vi "init.vi"(3 "Container State":T11, 4 "Previous State":variant, 5 "Previous Version":T10) -> (2 "Current State":T1={"current frame index"=0, "number of images"=0, "ROI (frames)"={"ROI"=[]}, "control refs"={"frame"=refnum, "image"=refnum, "saveROIsButton"=refnum, "loadImageSwitch"=refnum, "loadROIsSwitch"=refnum, "saveROIsSwitch"=refnum, "loadImagePath"=refnum, "loadROIPath"=refnum, "redraw"=refnum}, "calibration"={"x"=0.0, "y"=0.0, "x unit"=enum."um", "y unit"=enum."um"}, "xpaths"={"x offset"="", "y offset"="", "z offset"=""}, "offset"=refnum, "XML description"="", "number of ROIs"=0.0, "ROI Tool Buttons Visible"={"Zoom Tool"=FALSE, "Selection Tool"=FALSE, "Pan Tool"=FALSE, "Point Tool"=FALSE, "Line Tool"=FALSE, "Rectangle Tool"=FALSE, "Rotated Rectangle Tool"=FALSE, "Polyline Tool"=FALSE, "Polygon Tool"=FALSE, "Freehand Tool"=FALSE, "Closed Freehand Tool"=FALSE, "Ellipse Tool"=FALSE, "Annulus Tool"=FALSE}, "ROI color"=0, "number color"=0, "enable ROI numbering?"=FALSE, "selected path to save ROIs"=path "", "starting path"=path "", "array of overlays"=[], "pointCollection"=refnum, "ROImode"=enum."IMAQROIs", "selected point ID"=0.0, "point radius"=5, "point colours"=[], "PlotAreaSize"={"Width"=0, "Height"=0}, "last action"=enum."not specified"} {"array of overlays"."overlay size" min=1})   [LabVIEW 2010, in "XImage.xctl"]
uses:
  XImage.xctl
  state.ctl
  classes/SpaceVector/SpaceVector/SpaceVector.lvclass
  classes/PointCollection/PointCollection/PointCollection.lvclass
  ROI_frames_cluster.ctl
  control_refs_cluster.ctl
  calibration_cluster.ctl
  enumerations/unit.ctl
  xpath_cluster.ctl
  overlays_cluster.ctl
  ROI_mode_enum.ctl
  last_action_enum.ctl
  <vilib>/_xctls/Container State.ctl
  <vilib>/_xctls/Version.ctl
  <vilib>/_xctls/XControlSupport.lvlib
  classes/Image/Image/Image.lvclass
panel:
  in  "Default Indicator State":T1={"current frame index"=0, "number of images"=0, "ROI (frames)"={"ROI"=[]}, "control refs"={"frame"=refnum, "image"=refnum, "saveROIsButton"=refnum, "loadImageSwitch"=refnum, "loadROIsSwitch"=refnum, "saveROIsSwitch"=refnum, "loadImagePath"=refnum, "loadROIPath"=refnum, "redraw"=refnum}, "calibration"={"x"=0.0, "y"=0.0, "x unit"=enum."um", "y unit"=enum."um"}, "xpaths"={"x offset"="", "y offset"="", "z offset"=""}, "offset"=refnum, "XML description"="", "number of ROIs"=0.0, "ROI Tool Buttons Visible"={"Zoom Tool"=FALSE, "Selection Tool"=FALSE, "Pan Tool"=FALSE, "Point Tool"=FALSE, "Line Tool"=FALSE, "Rectangle Tool"=FALSE, "Rotated Rectangle Tool"=FALSE, "Polyline Tool"=FALSE, "Polygon Tool"=FALSE, "Freehand Tool"=FALSE, "Closed Freehand Tool"=FALSE, "Ellipse Tool"=FALSE, "Annulus Tool"=FALSE}, "ROI color"=0, "number color"=0, "enable ROI numbering?"=FALSE, "selected path to save ROIs"=path "", "starting path"=path "", "array of overlays"=[], "pointCollection"=refnum, "ROImode"=enum."IMAQROIs", "selected point ID"=0.0, "point radius"=5, "point colours"=[], "PlotAreaSize"={"Width"=0, "Height"=0}, "last action"=enum."not specified"} {"array of overlays"."overlay size" min=1}
  in  "Default Control State":T1={"current frame index"=0, "number of images"=0, "ROI (frames)"={"ROI"=[]}, "control refs"={"frame"=refnum, "image"=refnum, "saveROIsButton"=refnum, "loadImageSwitch"=refnum, "loadROIsSwitch"=refnum, "saveROIsSwitch"=refnum, "loadImagePath"=refnum, "loadROIPath"=refnum, "redraw"=refnum}, "calibration"={"x"=0.0, "y"=0.0, "x unit"=enum."um", "y unit"=enum."um"}, "xpaths"={"x offset"="", "y offset"="", "z offset"=""}, "offset"=refnum, "XML description"="", "number of ROIs"=0.0, "ROI Tool Buttons Visible"={"Zoom Tool"=FALSE, "Selection Tool"=FALSE, "Pan Tool"=FALSE, "Point Tool"=FALSE, "Line Tool"=FALSE, "Rectangle Tool"=FALSE, "Rotated Rectangle Tool"=FALSE, "Polyline Tool"=FALSE, "Polygon Tool"=FALSE, "Freehand Tool"=FALSE, "Closed Freehand Tool"=FALSE, "Ellipse Tool"=FALSE, "Annulus Tool"=FALSE}, "ROI color"=0, "number color"=0, "enable ROI numbering?"=FALSE, "selected path to save ROIs"=path "", "starting path"=path "", "array of overlays"=[], "pointCollection"=refnum, "ROImode"=enum."IMAQROIs", "selected point ID"=0.0, "point radius"=5, "point colours"=[], "PlotAreaSize"={"Width"=0, "Height"=0}, "last action"=enum."not specified"} {"array of overlays"."overlay size" min=1}
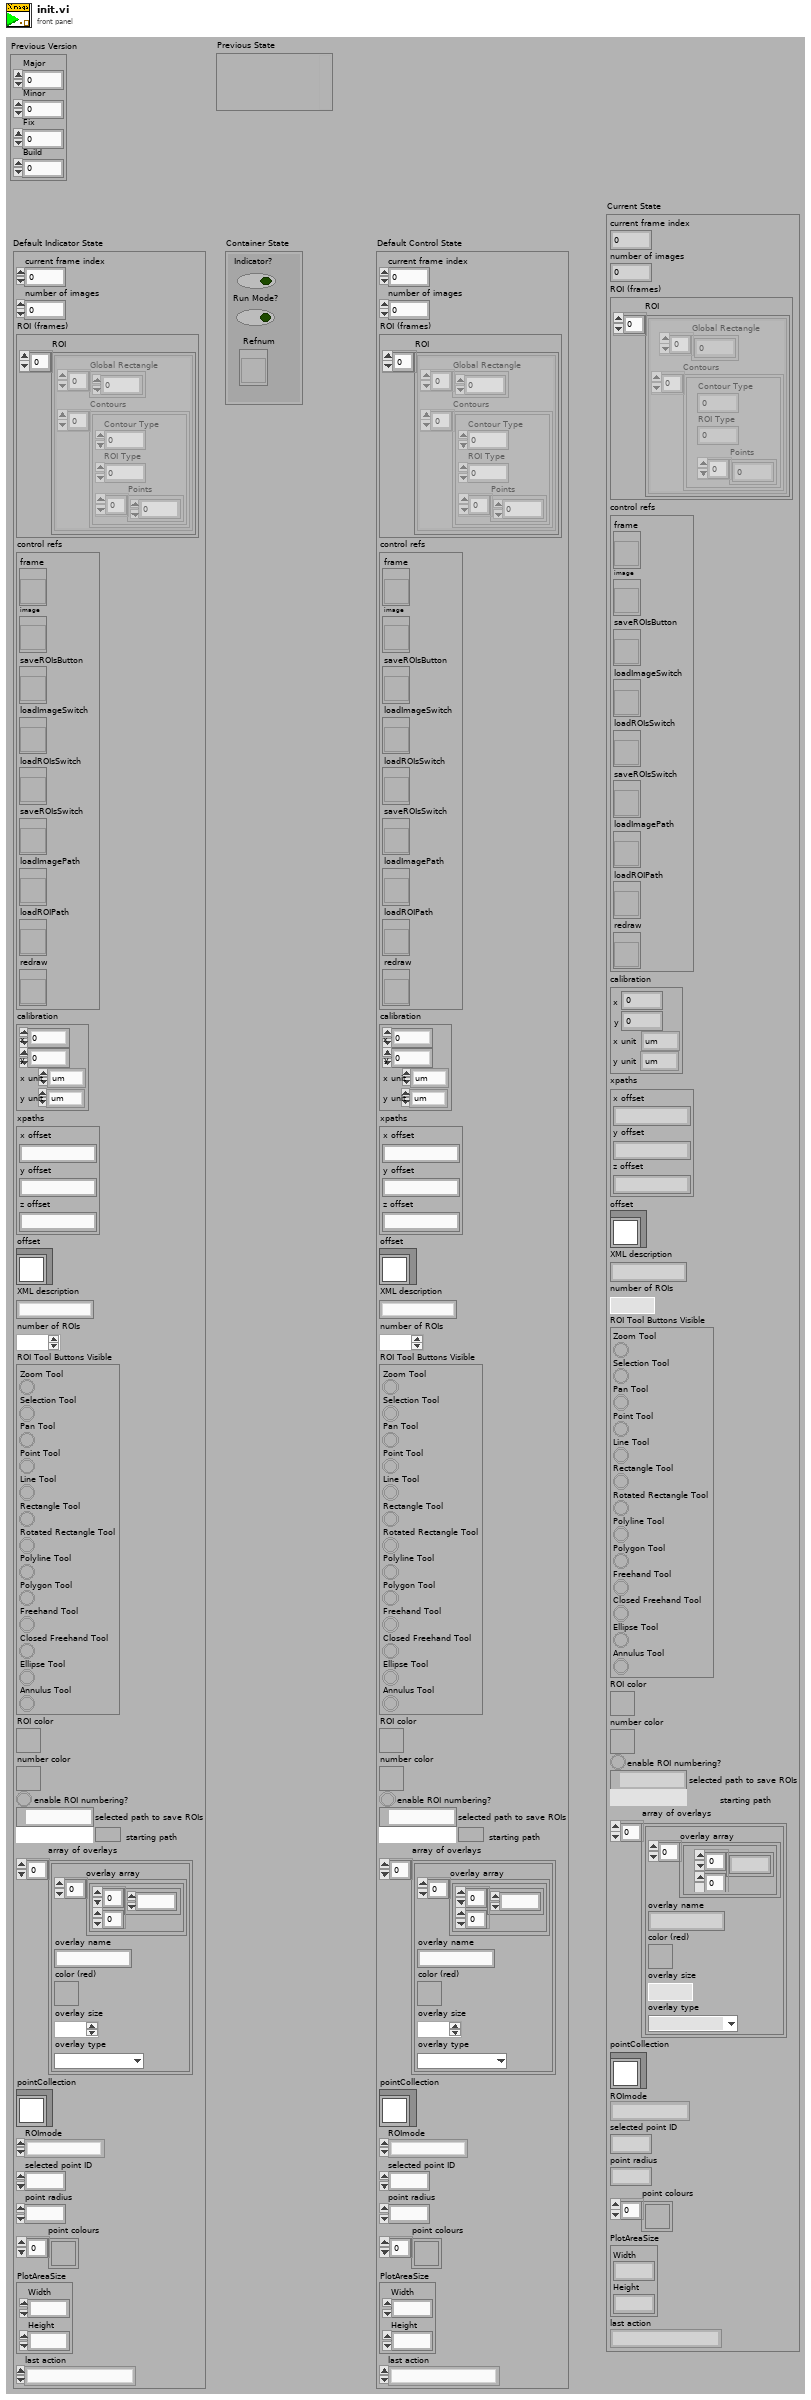
[diagram p1: front panel]
types:
  T1 = typedef "XImage.xctl/state.ctl" = cluster{"current frame index":i32, "number of images":i32, "ROI (frames)":T2, "control refs":T3, "calibration":T4, "xpaths":T6, "offset":refnum<class "SpaceVector.lvclass">, "XML description":string, "number of ROIs":dbl, "ROI Tool Buttons Visible":cluster{"Zoom Tool":bool, "Selection Tool":bool, "Pan Tool":bool, "Point Tool":bool, "Line Tool":bool, "Rectangle Tool":bool, "Rotated Rectangle Tool":bool, "Polyline Tool":bool, "Polygon Tool":bool, "Freehand Tool":bool, "Closed Freehand Tool":bool, "Ellipse Tool":bool, "Annulus Tool":bool}, "ROI color":u32, "number color":u32, "enable ROI numbering?":bool, "selected path to save ROIs":path, "starting path":path, "array of overlays":T7[], "pointCollection":refnum<class "PointCollection.lvclass">, "ROImode":T8, "selected point ID":dbl, "point radius":i32, "point colours":u32[], "PlotAreaSize":cluster{"Width":u32, "Height":u32}, "last action":T9}
  T2 = typedef "XImage.xctl/ROI_frames_cluster.ctl" = cluster{"ROI":cluster{"Global Rectangle":i32[], "Contours":cluster{"Contour Type":u32, "ROI Type":u32, "Points":i32[]}[]}[]}
  T3 = typedef "XImage.xctl/control_refs_cluster.ctl" = cluster{"frame":refnum<vi>, "image":refnum<vi>, "saveROIsButton":refnum<vi>, "loadImageSwitch":refnum<vi>, "loadROIsSwitch":refnum<vi>, "saveROIsSwitch":refnum<vi>, "loadImagePath":refnum<vi>, "loadROIPath":refnum<vi>, "redraw":refnum<vi>}
  T4 = typedef "XImage.xctl/calibration_cluster.ctl" = cluster{"x":dbl, "y":dbl, "x unit":T5, "y unit":T5}
  T5 = typedef "Image.lvclass/unit.ctl" = enum16{"um", "s"}
  T6 = typedef "XImage.xctl/xpath_cluster.ctl" = cluster{"x offset":string, "y offset":string, "z offset":string}
  T7 = typedef "XImage.xctl/overlays_cluster.ctl" = cluster{"overlay array":cluster{i32[][]}[], "overlay name":string, "color (red)":u32, "overlay size":i32, "overlay type":enum16{"crosshair", "circle"}}
  T8 = typedef "XImage.xctl/ROI_mode_enum.ctl" = enum16{"none", "IMAQROIs", "PointCollection"}
  T9 = typedef "XImage.xctl/last_action_enum.ctl" = enum16{"not specified", "image loaded", "frame changed", "ROIs changed"}
  T10 = typedef "XControlSupport.lvlib/Version.ctl" = cluster{"Major":u16, "Minor":u16, "Fix":u16, "Build":u16}
  T11 = typedef "XControlSupport.lvlib/Container State.ctl" = cluster{"Indicator?":bool, "Run Mode?":bool, " Refnum":refnum<vi>}
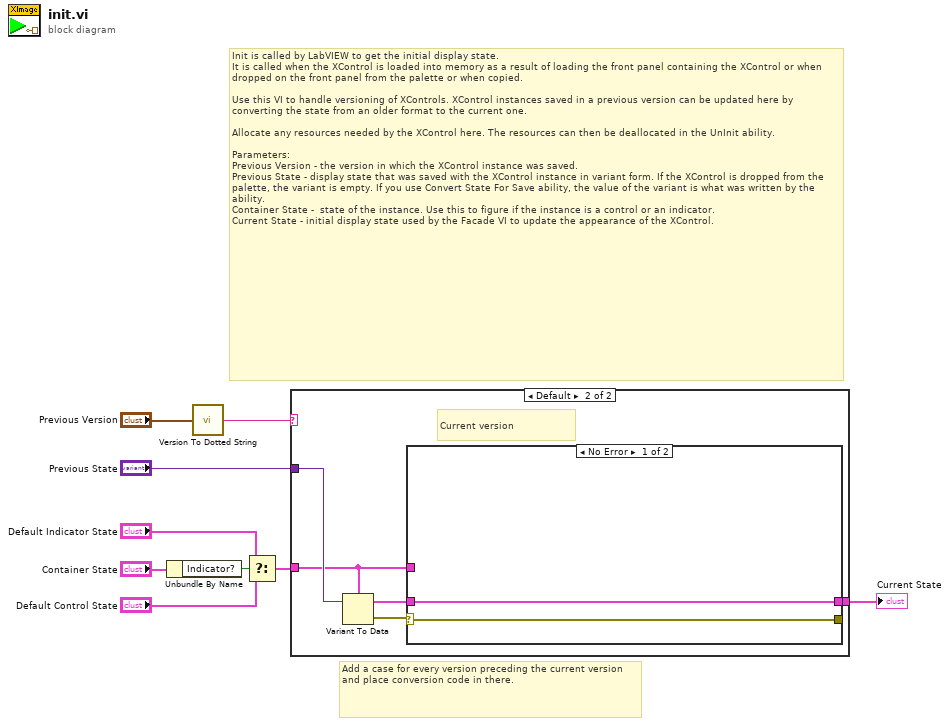
[diagram p0: block diagram]
diagram:
  # "Add a case for every version preceding the current version and place conversion code in there."
  # "Init is called by LabVIEW to get the initial display state.\nIt is called when the XControl is loaded into memory as a result of loading the front panel containing the XControl or when dropped on the front panel from the palette or when copied.\n\nUse this VI to handle versioning of XControls. XControl instances saved in a previous version can be updated here by converting the state from an older format to the current one.\n\nAllocate any resources needed by the XControl here. The resources can then be deallocated in the UnInit ability.\n\nParameters:\nPrevious Version - the version in which the XControl instance was saved.\nPrevious State - display state that was saved with the XControl instance in variant form. If the XControl is dropped from the palette, the variant is empty. If you use Convert State For Save ability, the value of the variant is what was written by the ability. \nContainer State -  state of the instance. Use this to figure if the instance is a control or an indicator.\nCurrent State - initial display state used by the Facade VI to update the appearance of the XControl."
  n1 = Unbundle By Name("Container State") -> ("Indicator?"=w4:bool)
  n2 = call <vilib>:"Version To Dotted String.vi"("Version"="Previous Version") -> ("String Version"=w1:string)
  n3 = Select(t="Default Indicator State", s=w4, f="Default Control State") -> (s? t:f=w3:T1)
  n4 = case shown="Default" w1 {
    tunnel: "Previous State" -> [_ w15]
    tunnel: [w10 w11] -> w8
    tunnel: w3 -> [w10 w12]
    frame "0.0.0.0" {
      # "Just created, use default state"
    }
    frame Default {
      # "Current version"
      n5 = Variant To Data(Variant=w15, type=w12) -> (error out=w14:errorcluster, data=w13:T1)  [unwired: 1 in]
      n6 = case shown="No Error" w14 {
        selector: w14 -> [w17 w18]
        tunnel: w13 -> [w16 _]
        tunnel: [w16 w19] -> w11
        tunnel: w12 -> [_ w19]
        tunnel: [w17 w18] -> _
        frame No Error {
        }
        frame Error {
          # "Error converting previously \nsaved state. Use default instead."
        }
      }
    }
  }
  "Current State" <- w8
